vi "Get_Install_Path.vi"(8 "error in (no error)":errorcluster, 10 "IB_Source in":refnum<class "IB_Source.lvclass">, 11 "IB_Tree_Item_Source_Folder in":refnum<class "IB_Tree_Item_Source_Folder.lvclass">) -> (0 "error out":errorcluster, 2 "eng_installPath":string, 3 "IB_Tree_Item_Source_Folder out":refnum<class "IB_Tree_Item_Source_Folder.lvclass">)   [LabVIEW 2020, in "IB_Tree_Item_Source_Folder.lvclass"]
uses:
  <vilib>/AppBuilder/IB_Classes/Tree_Item_Source_Folder/IB_Tree_Item_Source_Folder.lvclass
  <vilib>/AppBuilder/IB_Classes/Tree_Item_Source_Folder/IB_Tree_Item_Source_Folder.lvclass/IB_Tree_Item_Source_Folder.ctl
  <vilib>/AppBuilder/IB_Classes/Source/IB_Source.lvclass
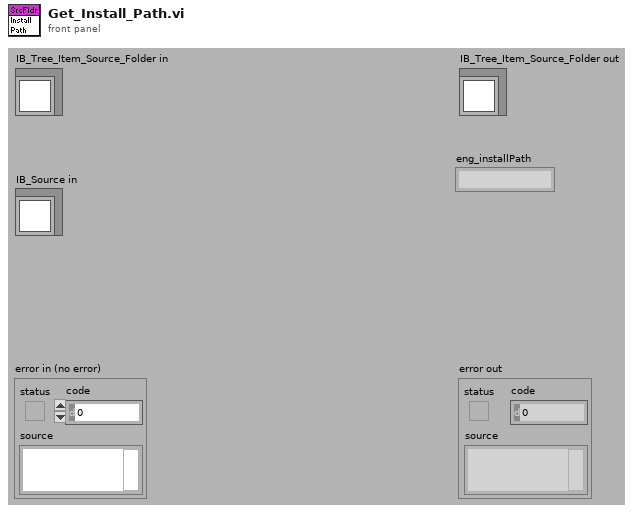
[diagram p1: front panel]
types:
  T1 = typedef "IB_Source.ctl" = cluster{"name":string, "sourceTag":string, "destTag":string, "path":path, "eng_installPath":string, "UI_inBuild?":bool, "str ref?":bool}
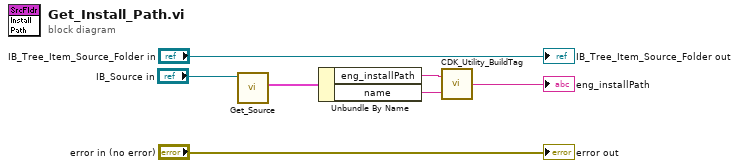
[diagram p0: block diagram]
diagram:
  n1 = call <vilib>:"Get_Source.vi"("IB_Source in"="IB_Source in") -> ("data"=w7:T1)  [unwired: 1 in, 9 out]
  n2 = Unbundle By Name(w7) -> ("eng_installPath"=w6:string, "name"=w5:string)
  n3 = call <resource>:"CDK_Utility_BuildTag.vi"("name or relative path"=w5, "BasePath"=w6) -> ("appended path"=→"eng_installPath":string)
  "error out" <- "error in (no error)"
  "IB_Tree_Item_Source_Folder out" <- "IB_Tree_Item_Source_Folder in"
